vi "VISA IO.vi"(7 "write buffer":string, 8 "error in (no error)":errorcluster, 11 "VISA resource name":refnum<visa-resource-name>="TCPIP0::localhost::hislip1::INSTR") -> (0 "error out":errorcluster, 3 "read buffer":string)   [LabVIEW 2020]
doc: "abce"
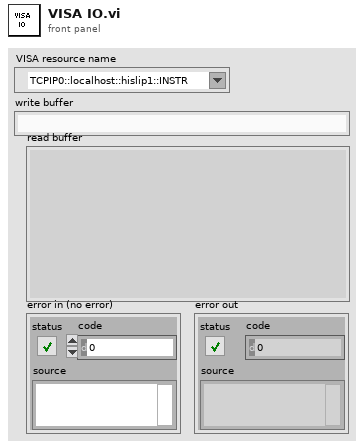
[diagram p1: front panel]
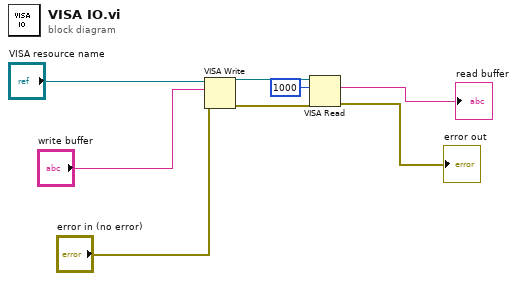
[diagram p0: block diagram]
diagram:
  n1 = VISA Write(VISA resource name="VISA resource name", write buffer="write buffer", error in (no error)="error in (no error)") -> (VISA resource name out=w6:refnum<visa-resource-name>, error out=w5:errorcluster)  [unwired: 1 out]
  n2 = VISA Read(VISA resource name=w6, byte count=u32 1000, error in (no error)=w5) -> (read buffer=→"read buffer":string, error out=→"error out":errorcluster)  [unwired: 2 out]
